vi "Update Settings.vi"(8 "error in (no error)":errorcluster {"code" format="Error %.0f"}, 11 "Processing\nSettings In":T1={"Edlen\nSettings"={"P_atm"=100, "T (deg C)"=50, "PP h20"=100.0}, "Processing\nSettings"={"Subset Length"=100, "Peak Width"=50, "Filter Width"=100, "Threshold (V)"=1.0}} {"Processing\nSettings"."Threshold (V)" format="%0.2f"; "Edlen\nSettings"."PP h20" format="%0.2f"}) -> (0 "error out":errorcluster {"code" format="Error %.0f"}, 3 "Processing\nSettings Out":T1={"Edlen\nSettings"={"P_atm"=100, "T (deg C)"=50, "PP h20"=100.0}, "Processing\nSettings"={"Subset Length"=100, "Peak Width"=50, "Filter Width"=100, "Threshold (V)"=1.0}} {"Processing\nSettings"."Threshold (V)" format="%0.2f"; "Edlen\nSettings"."PP h20" format="%0.2f"})   [LabVIEW 2018]
uses:
  Type Defs/Processing Settings 1.ctl
panel:
  in  "Processing\nSettings":T1={"Edlen\nSettings"={"P_atm"=100, "T (deg C)"=50, "PP h20"=100.0}, "Processing\nSettings"={"Subset Length"=100, "Peak Width"=50, "Filter Width"=100, "Threshold (V)"=1.0}} {"Processing\nSettings"."Threshold (V)" format="%0.2f"; "Edlen\nSettings"."PP h20" format="%0.2f"}
  in  "Cancel Button":bool
  in  "OK Button":bool
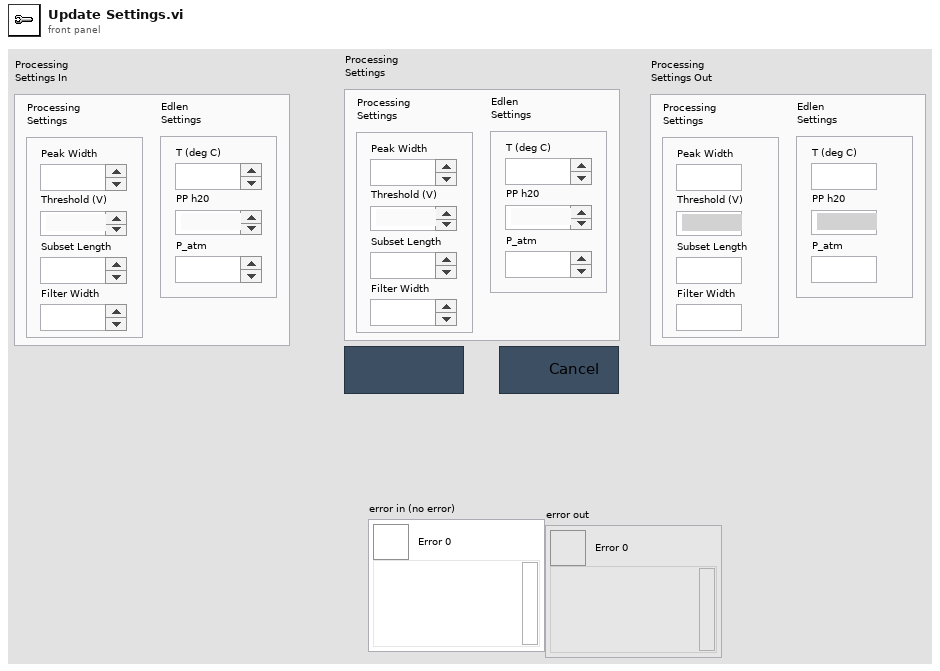
[diagram p1: front panel]
types:
  T1 = typedef "Processing Settings 1.ctl" = cluster{"Edlen\nSettings":cluster{"P_atm":i32, "T (deg C)":i32, "PP h20":dbl}, "Processing\nSettings":cluster{"Subset Length":i32, "Peak Width":i32, "Filter Width":i32, "Threshold (V)":dbl}}
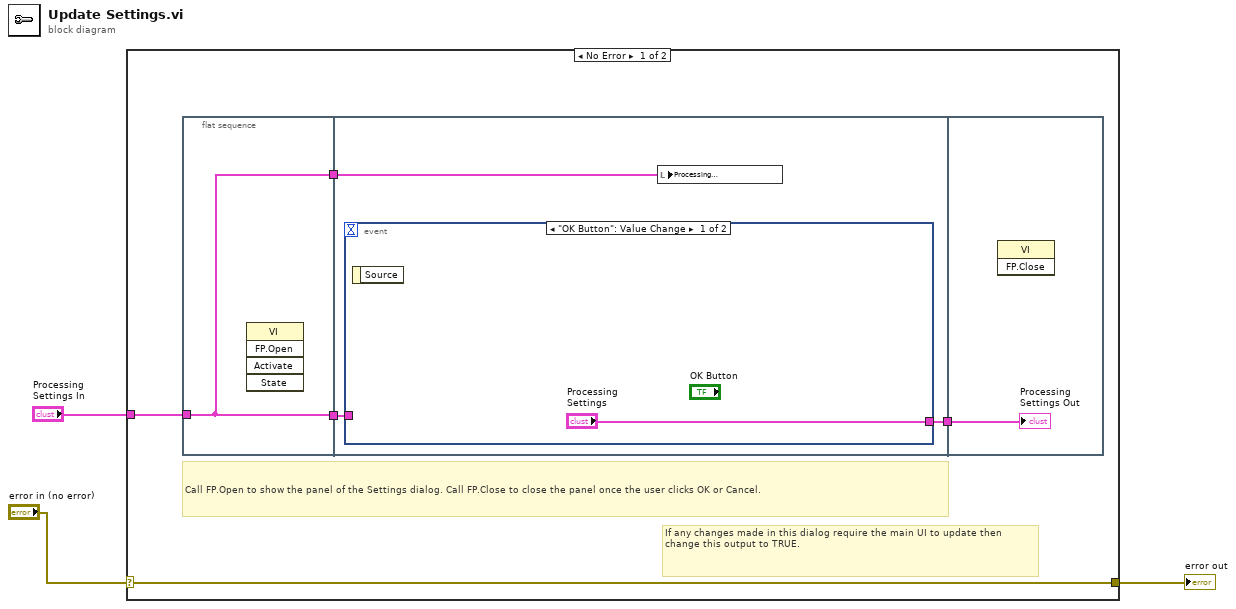
[diagram p0: block diagram]
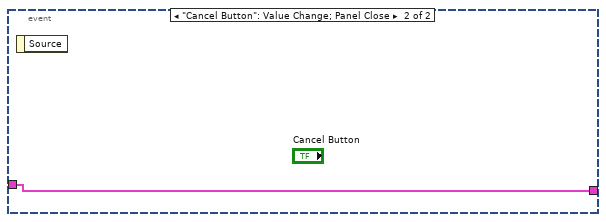
[diagram p2: hidden frame]
diagram:
  n1 = case shown="No Error" "error in (no error)" {
    selector: "error in (no error)" -> [w8 w16]
    tunnel: [w8 w16] -> w2
    tunnel: "Processing\nSettings In" -> [w5 _]
    frame No Error {
      # "Call FP.Open to show the panel of the Settings dialog. Call FP.Close to close the panel once the user clicks OK or Cancel."
      # "If any changes made in this dialog require the main UI to update then change this output to TRUE."
      n2 = flat-sequence {
        tunnel: [w9] -> w6
        tunnel: w5 -> [w9]
        tunnel: [w9] -> w4
        tunnel: [w12] -> w7
        tunnel: w6 -> [w11]
        tunnel: w4 -> [w10]
        tunnel: w7 -> [w15]
        frame #0 {
          n3 = invoke class="VI" method="FP.Open"() -> ()  [unwired: 5 in, 5 out]
        }
        frame #1 {
          n4 = event shown="[0] \"OK Button\": Value Change" {
            selector: _ -> [_ _]
            dyn-events: _ -> [_ _]
            timeout: _ -> [_ _]
            tunnel: ["Processing\nSettings" w14] -> w12
            tunnel: w11 -> [_ w14]
            event "OK Button": Value Change {
              n5 = event-data() -> ()  [unwired: 1 in, 1 out]
            }
            event "Cancel Button": Value Change; Panel Close {
              n6 = event-data() -> ()  [unwired: 1 in, 1 out]
            }
          }
          n7 = local write "Processing\nSettings"(w10) -> ()
        }
        frame #2 {
          n8 = invoke class="VI" method="FP.Close"() -> ()  [unwired: 3 in, 3 out]
          "Processing\nSettings Out" <- w15
        }
      }
    }
    frame Error {
    }
  }
  "error out" <- w2
